vi "2 mission_interpreter.vi"(9 "Move to Front?":bool, 11 "Mission.lvclass":refnum<class "Mission.lvclass">) -> ()   [LabVIEW 2011]
uses:
  2 Classes/Waypoint/Waypoint.lvclass
  2 Classes/Mission/Mission.lvclass
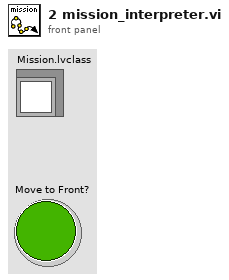
[diagram p1: front panel]
types:
  T1 = enum16{"Round Buoy", "Pass Buoys", "Station Keeping"}
  T2 = typedef "UTM Location.ctl" = cluster{"UTM Zone":dbl, "Hemisphere":enum16{"North", "South"}, "East":dbl, "North":dbl}
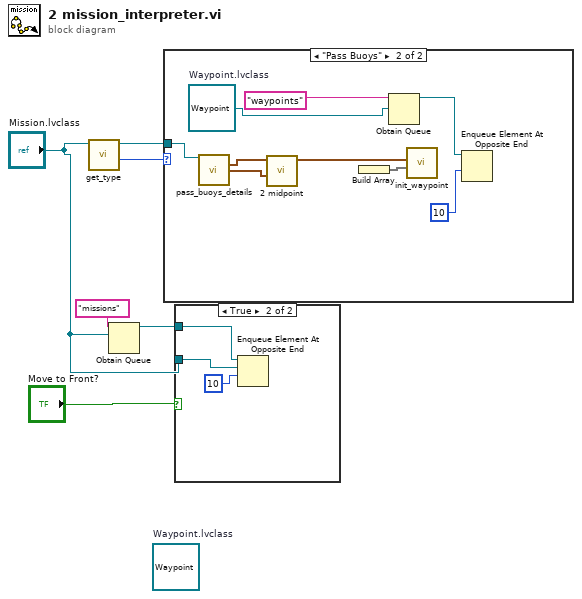
[diagram p0: block diagram]
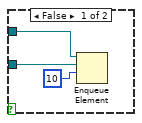
[diagram p3: hidden frame]
diagram:
  (unwired) refnum<class "Waypoint.lvclass"> refnum  # Waypoint.lvclass
  n1 = call-dynamic "get_type.vi"("Mission in"="Mission.lvclass") -> ("Enum"=w3:T1, "Mission out"=w2:refnum<class "Mission.lvclass">)  [unwired: 8 in, 1 out]
  n2 = Obtain Queue(name (unnamed)="missions", element data type="Mission.lvclass") -> (queue out=w1:refnum<queue>)  [unwired: 3 in, 2 out]
  n3 = case shown="\"Pass Buoys\"" w3 {
    tunnel: w2 -> [_ w15]
    frame "Round Buoy", Default {
    }
    frame "Pass Buoys" {
      w11 = refnum<class "Waypoint.lvclass"> refnum  # Waypoint.lvclass
      n4 = call-dynamic "pass_buoys_details.vi"("Mission in"=w15) -> ("Buoy Pass 1"=w14:T2, "Buoy Pass 2"=w13:T2)  [unwired: 11 in, 2 out]
      n5 = call "2 midpoint.vi"("UTM 2"=w13, "UTM 1"=w14) -> ("Midpoint"=w8:T2)  [unwired: 9 in]
      n6 = Build Array() -> (w7:void[])  [unwired: 1 in]
      n7 = Obtain Queue(name (unnamed)="waypoints", element data type=w11) -> (queue out=w9:refnum<queue>)  [unwired: 3 in, 2 out]
      n8 = call "init_waypoint.vi"("No Sail Circles"=w7, "Coords"=w8) -> ()  [unwired: 9 in, 1 out]
      n9 = Enqueue Element At Opposite End(queue=w9, timeout in ms (-1)=10) -> ()  [unwired: 2 in, 3 out]
    }
  }
  n10 = case shown="True" "Move to Front?" {
    tunnel: w1 -> [w18 w21]
    tunnel: "Mission.lvclass" -> [w17 w20]
    frame False {
      n11 = Enqueue Element(queue=w18, element=w17, timeout in ms (-1)=10) -> ()  [unwired: 1 in, 3 out]
    }
    frame True {
      n12 = Enqueue Element At Opposite End(queue=w21, element=w20, timeout in ms (-1)=10) -> ()  [unwired: 1 in, 3 out]
    }
  }
